vi "Check Output Result.vi"(7 "Execution in":refnum<data-value>, 8 "Output Values":cluster{"Name":string, "Variant Data":variant}[](array[cluster]), 11 "Step Output":T5) -> (2 "Measure Result":T1, 3 "Include In Result":bool, 5 "Execution out":refnum<data-value>)   [LabVIEW 2015, in "Execution.lvclass"]
uses:
  Execution.lvclass
  Step/STEP_OUTPUT.ctl
  Step/OUTPUT_DATA_TYPE.ctl
  OutputUI/OUTPUT_CHECK_TYPE.ctl
  Step/OUTPUT_VALUE_TYPE.ctl
  STEP_MEASURE_RESULT.ctl
  Step/STEP_STATUS.ctl
  <vilib>/Utility/error.llb/DialogType.ctl
  Step.lvclass
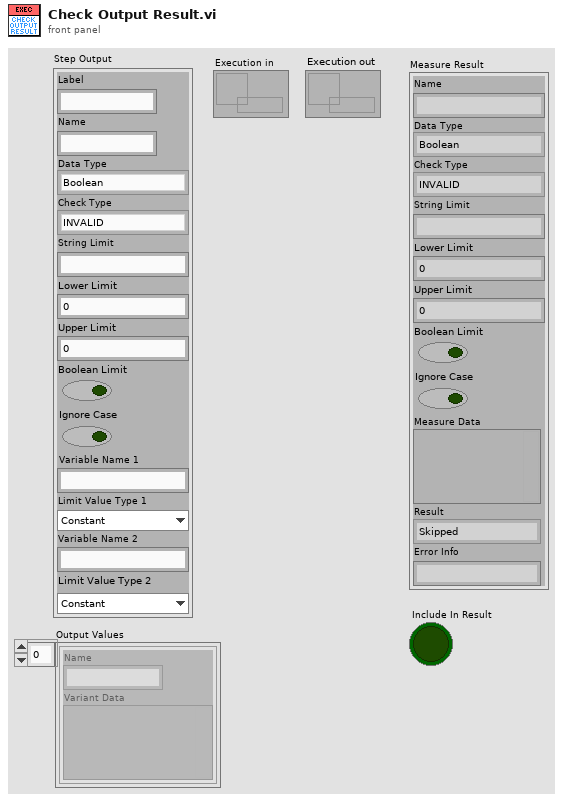
[diagram p1: front panel]
types:
  T1 = typedef "Execution.lvclass/STEP_MEASURE_RESULT.ctl" = cluster{"Name":string, "Data Type":T2, "Check Type":T3, "String Limit":string, "Lower Limit":dbl, "Upper Limit":dbl, "Boolean Limit":bool, "Ignore Case":bool, "Measure Data":variant, "Result":T4, "Error Info":string}
  T2 = typedef "Step.lvclass/OUTPUT_DATA_TYPE.ctl" = enum16{"Boolean", "String", "Numeric", "Other"}
  T3 = typedef "Step.lvclass/OUTPUT_CHECK_TYPE.ctl" = enum16{"INVALID", "DO_NOT_CHECK", "RECORD", "VARIABLE", "EQUAL", "NOT_EQUAL", "STR_CONTAINS", "STR_START_WITH", "STR_END_WITH", "STR_REGEX_MATCH", "NUM_GT", "NUM_LT", "NUM_GE", "NUM_LE", "NUM_RANGE", "NUM_RANGE_BDY"}
  T4 = typedef "Step.lvclass/STEP_STATUS.ctl" = enum16{"Skipped", "Done", "Passed", "Failed", "Error"}
  T5 = typedef "Step.lvclass/STEP_OUTPUT.ctl" = cluster{"Label":string, "Name":string, "Data Type":T2, "Check Type":T3, "String Limit":string, "Lower Limit":dbl, "Upper Limit":dbl, "Boolean Limit":bool, "Ignore Case":bool, "Variable Name 1":string, "Limit Value Type 1":T6, "Variable Name 2":string, "Limit Value Type 2":T6}
  T6 = typedef "Step.lvclass/OUTPUT_VALUE_TYPE.ctl" = enum16{"Constant", "Variable"}
  T7 = typedef "DialogType.ctl" = u16
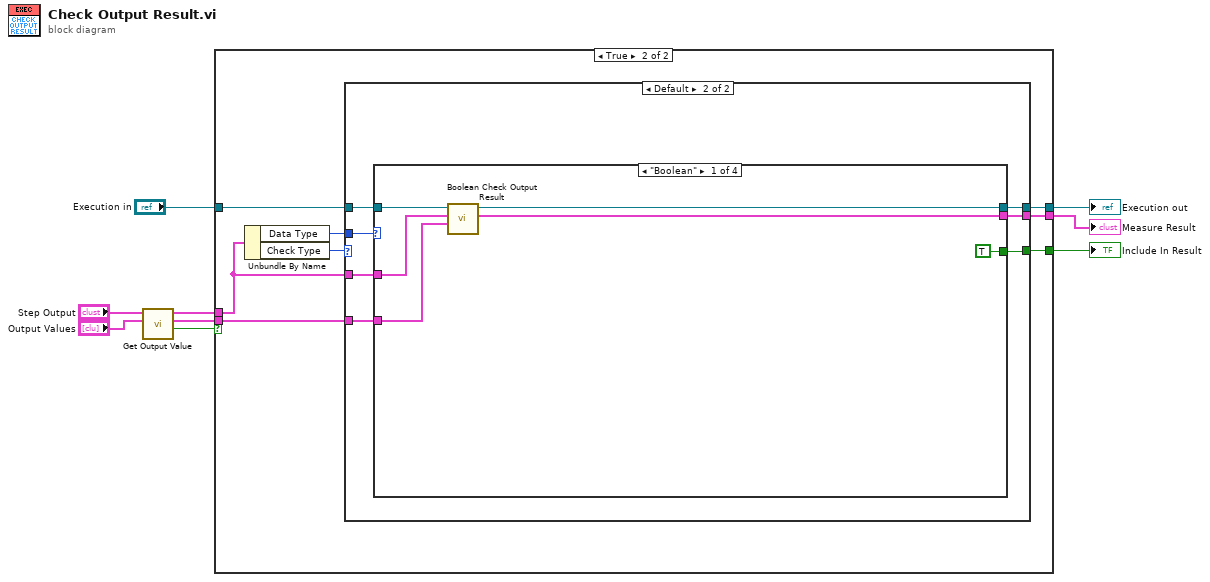
[diagram p0: block diagram]
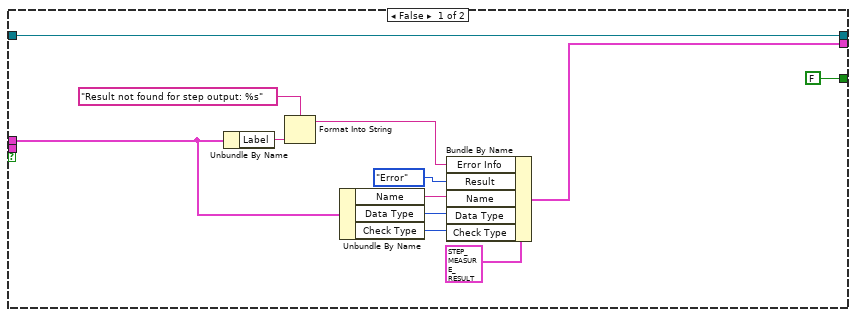
[diagram p2: hidden frame]
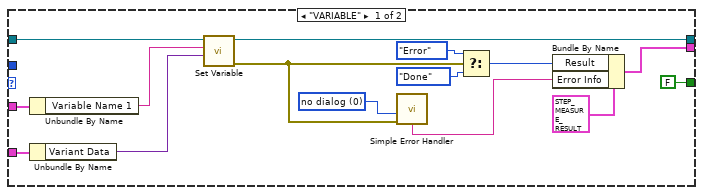
[diagram p3: hidden frame]
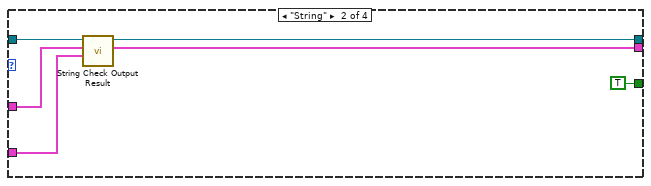
[diagram p4: hidden frame]
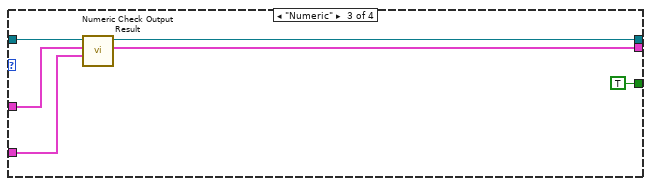
[diagram p5: hidden frame]
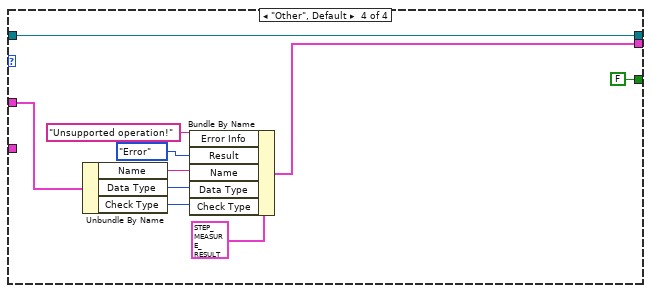
[diagram p6: hidden frame]
diagram:
  n1 = call "Get Output Value.vi"("Output Values"="Output Values", "Step Output in"="Step Output") -> ("Found"=w4:bool, "Output Value"=w3:cluster{"Name":string, "Variant Data":variant}, "Step Output out"=w5:T5)  [unwired: 7 in]
  n2 = case shown="True" w4 {
    tunnel: w3 -> [_ w29]
    tunnel: w5 -> [w17 w28]
    tunnel: "Execution in" -> [w19 w26]
    tunnel: [w19 w25] -> w6
    tunnel: [w11 w23] -> w2
    tunnel: [FALSE w22] -> w1
    frame False {
      n3 = Unbundle By Name(w17) -> ("Label"=w20:string)
      n4 = Format Into String(format string="Result not found for step output: %s", w20) -> (resulting string=w13:string)  [unwired: 2 in, 1 out]
      n5 = Unbundle By Name(w17) -> ("Name"=w16:string, "Data Type"=w15:T2, "Check Type"=w14:T3)
      n6 = Bundle By Name(cluster=T1 {"Name"="", "Data Type"=enum."Boolean", "Check Type"=enum."INVALID", "String Limit"="", "Lower Limit"=0.0, "Upper Limit"=0.0, "Boolean Limit"=FALSE, "Ignore Case"=FALSE, "Measure Data"=variant, "Result"=enum."Skipped", "Error Info"=""} ("Measure Result out"), "Error Info"=w13, "Result"=STEP_STATUS."Error" ("Status"), "Name"=w16, "Data Type"=w15, "Check Type"=w14) -> (w11:T1)
    }
    frame True {
      n7 = Unbundle By Name(w28) -> ("Data Type"=w24:T2, "Check Type"=w27:T3)
      n8 = case shown="Default" w27 {
        tunnel: w29 -> [w42 w48]
        tunnel: w28 -> [w44 w49]
        tunnel: w26 -> [w40 w50]
        tunnel: [w39 w47] -> w25
        tunnel: w24 -> [_ w51]
        tunnel: [w32 w46] -> w23
        tunnel: [FALSE w45] -> w22
        frame "VARIABLE" {
          w35 = T7 0 items=["no dialog", "OK message", "continue or stop message", "OK message + warnings", "continue/stop + warnings"] ("type of dialog (OK msg:1)")
          n9 = Unbundle By Name(w44) -> ("Variable Name 1"=w43:string)
          n10 = Unbundle By Name(w42) -> ("Variant Data"=w41:variant)
          n11 = call "Set Variable.vi"("Value"=w41, "Name"=w43, "Execution in"=w40) -> ("error out"=w36:errorcluster, "Execution out"=w39:refnum<data-value>)  [unwired: 7 in]
          n12 = call <vilib>:"Simple Error Handler.vi"("type of dialog (OK msg:1)"=w35, "error in (no error)"=w36) -> ("message"=w31:string)  [unwired: 3 in, 4 out]
          n13 = Select(t=STEP_STATUS."Error" ("Status"), s=w36, f=STEP_STATUS."Done" ("Status")) -> (s? t:f=w33:T4)
          n14 = Bundle By Name(cluster=T1 {"Name"="", "Data Type"=enum."Boolean", "Check Type"=enum."INVALID", "String Limit"="", "Lower Limit"=0.0, "Upper Limit"=0.0, "Boolean Limit"=FALSE, "Ignore Case"=FALSE, "Measure Data"=variant, "Result"=enum."Skipped", "Error Info"=""} ("Measure Result out"), "Result"=w33, "Error Info"=w31) -> (w32:T1)
        }
        frame Default {
          n15 = case shown="\"Boolean\"" w51 {
            tunnel: w50 -> [w57 w63 w69 w79]
            tunnel: w49 -> [w56 w62 w68 w72]
            tunnel: w48 -> [w55 w61 w67 _]
            tunnel: [w54 w60 w66 w79] -> w47
            tunnel: [w53 w59 w65 w70] -> w46
            tunnel: [TRUE TRUE TRUE FALSE] -> w45
            frame "Boolean" {
              n16 = call "Boolean Check Output Result.vi"("Output Value in"=w55, "Step Output in"=w56, "Execution in"=w57) -> ("Measure Result out"=w53:T1, "Execution out"=w54:refnum<data-value>)  [unwired: 7 in]
            }
            frame "String" {
              n17 = call "String Check Output Result.vi"("Output Value in"=w61, "Step Output in"=w62, "Execution in"=w63) -> ("Measure Result out"=w59:T1, "Execution out"=w60:refnum<data-value>)  [unwired: 7 in]
            }
            frame "Numeric" {
              n18 = call "Numeric Check Output Result.vi"("Output Value in"=w67, "Step Output in"=w68, "Execution in"=w69) -> ("Measure Result out"=w65:T1, "Execution out"=w66:refnum<data-value>)  [unwired: 7 in]
            }
            frame "Other", Default {
              n19 = Unbundle By Name(w72) -> ("Name"=w77:string, "Data Type"=w76:T2, "Check Type"=w75:T3)
              n20 = Bundle By Name(cluster=T1 {"Name"="", "Data Type"=enum."Boolean", "Check Type"=enum."INVALID", "String Limit"="", "Lower Limit"=0.0, "Upper Limit"=0.0, "Boolean Limit"=FALSE, "Ignore Case"=FALSE, "Measure Data"=variant, "Result"=enum."Skipped", "Error Info"=""} ("Measure Result out"), "Error Info"="Unsupported operation!", "Result"=STEP_STATUS."Error" ("Status"), "Name"=w77, "Data Type"=w76, "Check Type"=w75) -> (w70:T1)
            }
          }
        }
      }
    }
  }
  "Execution out" <- w6
  "Measure Result" <- w2
  "Include In Result" <- w1
